vi "MB Serial Init.vi"(4 "Timeout":u32=10000, 6 "Flow Control":u16(ring) items=["None", "XON/XOFF", "RTS/CTS", "XON/XOFF & RTS/CTS", "DTR/DSR", "XON/XOFF & DTR/DSR"], 7 "Mode":enum16{"RTU", "ASCII"}(ring), 8 "error in (no error)":errorcluster, 9 "Parity":u16(ring) items=["None", "Odd", "Even", "Mark", "Space"], 10 "Baud Rate":u32=9600, 11 "VISA resource name":refnum<visa-resource-name>) -> (0 "error out":errorcluster, 3 "VISA resource name out":refnum<visa-resource-name>)   [LabVIEW 2016]
doc: "Initializes the serial port specified by VISA resource name to the specified settings. Wire data to the VISA resource name input to determine the polymorphic instance to use or manually select the instance."
panel:
  # "VI Name: MB Serial Init.vi\nPurpose: Initializes the serial port for Modbus."
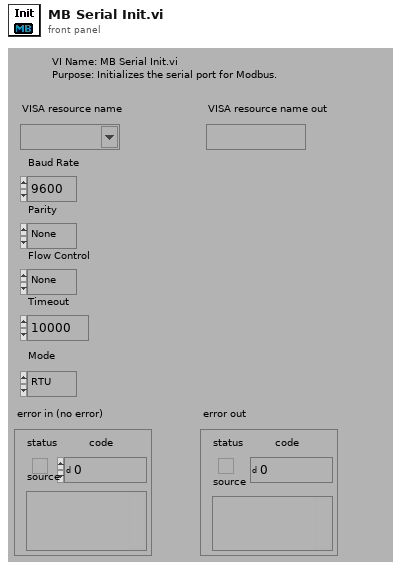
[diagram p1: front panel]
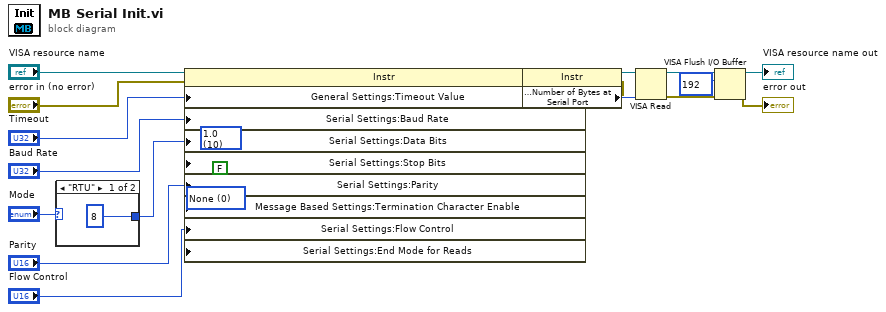
[diagram p0: block diagram]
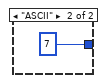
[diagram p2: hidden frame]
diagram:
  w18 = u16 0 items=["None", "LastBit", "TermChar"] ("Serial Settings:Serial End Mode for Reads")
  w20 = u16 10 items=["1.0"=10, "1.5"=15, "2.0"=20] ("Serial Settings:Serial Stop Bits")
  n1 = case shown="\"RTU\"" "Mode" {
    tunnel: [u16 8 ("data bits") u16 7 ("data bits")] -> w19
    frame "RTU" {
    }
    frame "ASCII" {
    }
  }
  n2 = property class="Instr"(reference="VISA resource name", error in="error in (no error)", "General Settings:Timeout Value"="Timeout", "Serial Settings:Baud Rate"="Baud Rate", "Serial Settings:Data Bits"=w19, "Serial Settings:Stop Bits"=w20, "Serial Settings:Parity"="Parity", "Message Based Settings:Termination Character Enable"=FALSE, "Serial Settings:Flow Control"="Flow Control", "Serial Settings:End Mode for Reads"=w18) -> (reference out=w9:refnum<visa-resource-name>, error out=w10:errorcluster)
  n3 = property class="Instr"(reference=w9, error in=w10) -> (reference out=w3:refnum<visa-resource-name>, error out=w1:errorcluster, "Serial Settings:Number of Bytes at Serial Port"=w2:u32)
  n4 = VISA Read(VISA resource name=w3, byte count=w2, error in (no error)=w1) -> (VISA resource name out=w4:refnum<visa-resource-name>, error out=w5:errorcluster)  [unwired: 2 out]
  n5 = VISA Flush I/O Buffer(VISA resource name=w4, mask (16)=u16 192, error in (no error)=w5) -> (VISA resource name out=→"VISA resource name out":refnum<visa-resource-name>, error out=→"error out":errorcluster)
